vi "TelnetClient.vi"() -> ()   [LabVIEW 2013]
doc: "The Telnet Line Client VI uses the Telnet VIs to simulate a simple Telnet Window."
uses:
  <vilib>/addons/internet/NI_InternetTK_Core_VIs.lvlib
panel:
  out "telnet error":errorcluster
  in  "echo":bool=TRUE
  in  "clear":bool
  in  "stop":bool
  in  "address":string="192.168.1.128"
  in  "port":i32=23
  in  "send":bool
  in  "input":string="0 1.000 1 -1.0000 0 100 100"
  out "terminal":string
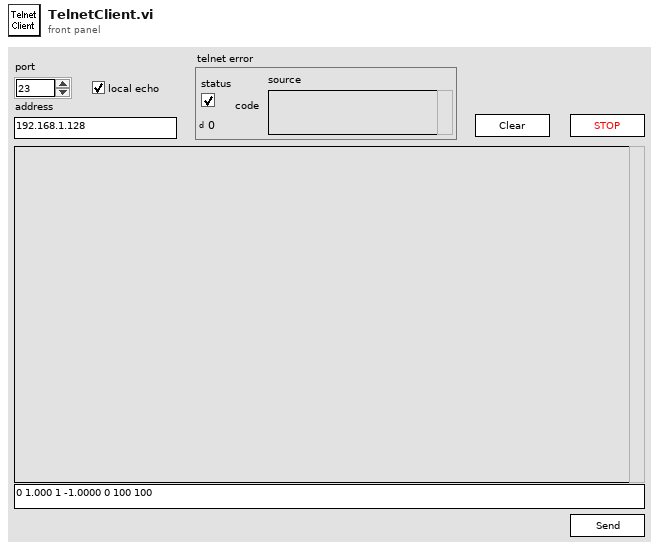
[diagram p1: front panel]
types:
  T1 = typedef "Telnet Session.ctl" = refnum<k1>
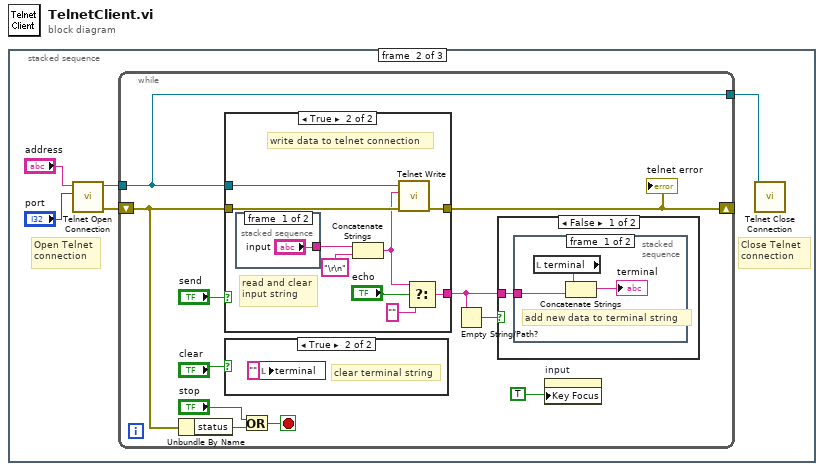
[diagram p0: block diagram]
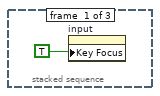
[diagram p2: hidden frame]
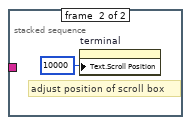
[diagram p3: hidden frame]
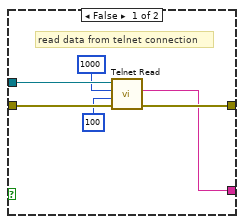
[diagram p5: hidden frame]
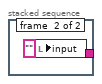
[diagram p6: hidden frame]
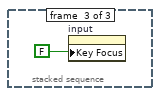
[diagram p8: hidden frame]
diagram:
  n1 = stacked-sequence {
    frame #0 {
      n2 = property on="input" class="Str"("Key Focus"=TRUE) -> ()  [unwired: 2 in, 2 out]
    }
    frame #1 {
      # "Close Telnet \nconnection"
      # "Open Telnet\nconnection"
      n3 = call <vilib>:"Telnet Open Connection.vi"("remote port (23)"="port", "address"="address") -> ("error out"=w3:errorcluster, "telnet connection"=w2:T1)  [unwired: 2 in, 6 out]
      n4 = while {
        shift-left: w3 -> [w9]
        shift-right: [w8] -> _
        tunnel: [w10] -> w4
        tunnel: w2 -> [w10]
        stop <- w15 stop-if-true
        n5 = Unbundle By Name(w9) -> ("status"=w13:bool)
        n6 = case shown="True" "send" {
          tunnel: [w25 w30] -> w12
          tunnel: w10 -> [w26 w37]
          tunnel: w9 -> [w28 w36]
          tunnel: [w27 w35] -> w8
          frame False {
            # "read data from telnet connection"
            n7 = call <vilib>:"Telnet Read.vi"("error in (no error)"=w28, "timeout ms (25000)"=100, "bytes to read"=1000, "telnet connection"=w26) -> ("error out"=w27:errorcluster, "data out"=w25:string)  [unwired: 4 out]
          }
          frame True {
            # "read and clear\ninput string"
            # "write data to telnet connection"
            n8 = stacked-sequence {
              tunnel: ["input" _] -> w34
              frame #0 {
              }
              frame #1 {
                n9 = local write "input"("" ("input")) -> ()
              }
            }
            n10 = Concatenate Strings(w34, "\r\n") -> (w29:string)
            n11 = call <vilib>:"Telnet Write.vi"("error in (no error)"=w36, "data in"=w29, "telnet connection"=w37) -> ("error out"=w35:errorcluster)  [unwired: 1 in, 5 out]
            n12 = Select(t=w29, s="echo", f="" ("data out")) -> (s? t:f=w30:string)
          }
        }
        "telnet error" <- w8
        n13 = case shown="True" "clear" {
          frame False {
          }
          frame True {
            # "clear terminal string"
            n14 = local write "terminal"("" ("terminal")) -> ()
          }
        }
        n15 = Or(x="stop", y=w13) -> (x .or. y?=w15:bool)
        n16 = Empty String/Path?(string/path=w12) -> (empty?=w11:bool)
        n17 = case shown="False" w11 {
          tunnel: w12 -> [w18 _]
          frame False {
            n18 = stacked-sequence {
              tunnel: w18 -> [w19 _]
              frame #0 {
                # "add new data to terminal string"
                n19 = local read "terminal"() -> (w20:string)
                n20 = Concatenate Strings(w20, w19) -> (→"terminal":string)
              }
              frame #1 {
                # "adjust position of scroll box"
                n21 = property on="terminal" class="Str"("Text.Scroll Position"=u32 10000 ("Scroll Position")) -> ()  [unwired: 2 in, 2 out]
              }
            }
          }
          frame True {
            # "input string empty"
          }
        }
        n22 = property on="input" class="Str"("Key Focus"=TRUE) -> ()  [unwired: 2 in, 2 out]
      }
      n23 = call <vilib>:"Telnet Close Connection.vi"("telnet connection"=w4) -> ()  [unwired: 1 in, 10 out]
    }
    frame #2 {
      n24 = property on="input" class="Str"("Key Focus"=FALSE) -> ()  [unwired: 2 in, 2 out]
    }
  }
